vi "SCLN_FindClientSlot.vi"(1 "Server Name":string) -> (0 "Client Index":i32)   [LabVIEW 2015]
uses:
  SCLN_INT32_Select.ctl
  SCLN_RW_Select.ctl
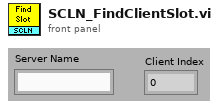
[diagram p1: front panel]
types:
  T1 = typedef "SCLN_RW_Select.ctl" = enum16{"Read", "Write"}
  T2 = typedef "SCLN_INT32_Select.ctl" = enum16{"Max_Servers", "Max_Clients", "Total_Servers", "Total_Clients"}
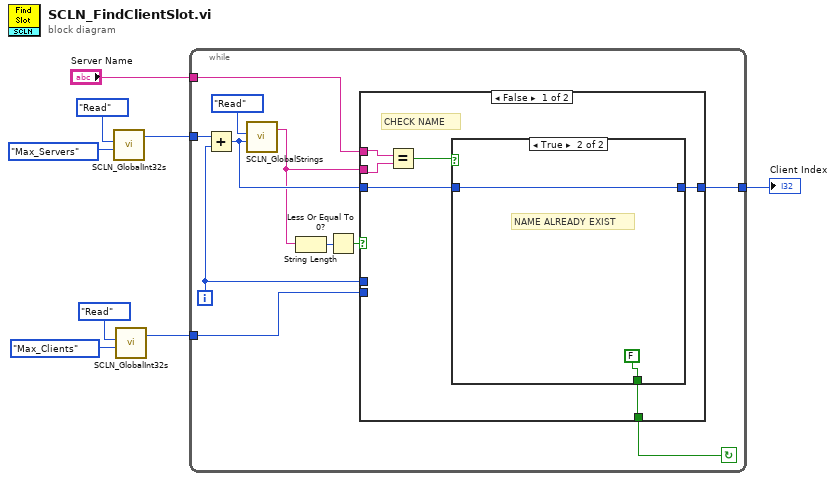
[diagram p0: block diagram]
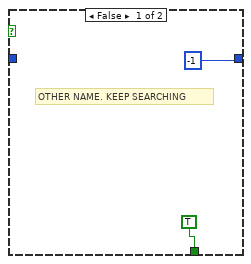
[diagram p2: hidden frame]
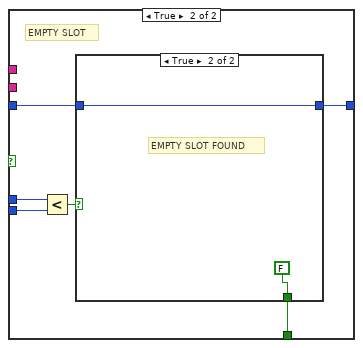
[diagram p3: hidden frame]
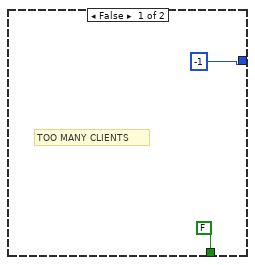
[diagram p4: hidden frame]
diagram:
  n1 = call "SCLN_GlobalInt32s.vi"("Element"=SCLN_INT32_Select."Max_Servers" ("GBL_INT32"), "Operation"=SCLN_RW_Select."Read" ("GBL_RW")) -> ("Read Value"=w4:i32)  [unwired: 2 in, 1 out]
  n2 = call "SCLN_GlobalInt32s.vi"("Element"=SCLN_INT32_Select."Max_Clients" ("GBL_INT32"), "Operation"=SCLN_RW_Select."Read" ("GBL_RW")) -> ("Read Value"=w3:i32)  [unwired: 2 in, 1 out]
  n3 = while {
    tunnel: w4 -> [w17]
    tunnel: w3 -> [w15]
    tunnel: [w12] -> w2
    tunnel: "Server Name" -> [w10]
    i -> [w14]
    stop <- w11 continue-if-true
    n4 = Add(x=w17, y=w14) -> (x+y=w13:i32)
    n5 = call "SCLN_GlobalStrings.vi"("Element"=w13, "Operation"=SCLN_RW_Select."Read" ("GBL_RW")) -> ("Read Value"=w9:string)  [unwired: 2 in, 1 out]
    n6 = String Length(string=w9) -> (length=w18:i32)
    n7 = Less Or Equal To 0?(x=w18) -> (x <= 0?=w16:bool)
    n8 = case shown="False" w16 {
      tunnel: w15 -> [_ w30]
      tunnel: w14 -> [_ w31]
      tunnel: w13 -> [w22 w34]
      tunnel: [w21 w33] -> w12
      tunnel: [w20 w32] -> w11
      tunnel: w10 -> [w24 _]
      tunnel: w9 -> [w25 _]
      frame False {
        # "CHECK NAME"
        n9 = Equal?(x=w24, y=w25) -> (x = y?=w23:bool)
        n10 = case shown="True" w23 {
          tunnel: w22 -> [_ w29]
          tunnel: [-1 w29] -> w21
          tunnel: [TRUE FALSE] -> w20
          frame False {
            # "OTHER NAME. KEEP SEARCHING"
          }
          frame True {
            # "NAME ALREADY EXIST"
          }
        }
      }
      frame True {
        # "EMPTY SLOT"
        n11 = Less?(x=w31, y=w30) -> (x < y?=w35:bool)
        n12 = case shown="True" w35 {
          tunnel: w34 -> [_ w39]
          tunnel: [-1 w39] -> w33
          tunnel: [FALSE FALSE] -> w32
          frame False {
            # "TOO MANY CLIENTS"
          }
          frame True {
            # "EMPTY SLOT FOUND"
          }
        }
      }
    }
  }
  "Client Index" <- w2
